vi "SubMark.vi"(0 "Refnum in":T1, 2 "Position Pixel":cluster{"x":sgl, "y":sgl}) -> ()   [LabVIEW 2015]
uses:
  <vilib>/vision/Image Controls.llb/IMAQ Image.ctl
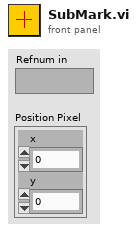
[diagram p1: front panel]
types:
  T1 = typedef "IMAQ Image.ctl" = refnum<image>
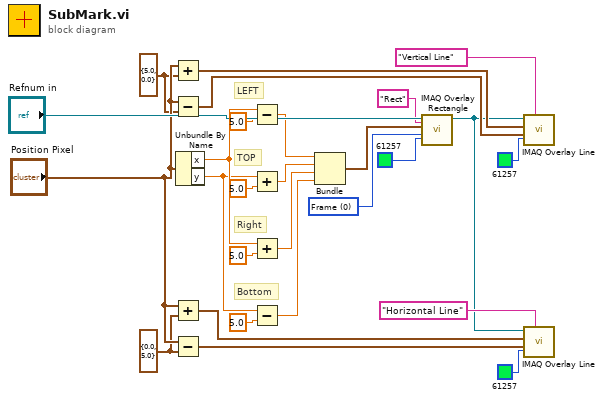
[diagram p0: block diagram]
diagram:
  w9 = cluster{"x":sgl, "y":sgl} {"x"=0.0, "y"=5.0} ("y")
  w14 = cluster{"x":sgl, "y":sgl} {"x"=5.0, "y"=0.0} ("y")
  w15 = u32 0 items=["Frame", "Fill", "Highlight"] ("Drawing Mode (Frame)")
  # "Bottom"
  # "Right"
  # "TOP"
  # "LEFT"
  n1 = Add(x="Position Pixel", y=w14) -> (x+y=w5:cluster{"x":sgl, "y":sgl})
  n2 = Subtract(x="Position Pixel", y=w14) -> (x-y=w13:cluster{"x":sgl, "y":sgl})
  n3 = Add(x="Position Pixel", y=w9) -> (x+y=w1:cluster{"x":sgl, "y":sgl})
  n4 = Subtract(x="Position Pixel", y=w9) -> (x-y=w8:cluster{"x":sgl, "y":sgl})
  n5 = Unbundle By Name("Position Pixel") -> ("x"=w3:sgl, "y"=w2:sgl)
  n6 = Subtract(x=w3, y=5.0) -> (x-y=w21:dbl)
  n7 = Add(x=w2, y=5.0) -> (x+y=w20:dbl)
  n8 = Add(x=w3, y=5.0) -> (x+y=w19:dbl)
  n9 = Subtract(x=w2, y=5.0) -> (x-y=w18:dbl)
  n10 = Bundle(w21, w20, w19, w18) -> (w17:cluster{dbl, dbl, dbl, dbl})  [unwired: 1 in]
  n11 = call "IMAQ Overlay Rectangle"("Color"=u32 61257, "Group"="Rect", "Drawing Mode (Frame)"=w15, "Rectangle"=w17, "Image"="Refnum in") -> ("Image Out"=w4:T1)  [unwired: 5 in, 1 out]
  n12 = call "IMAQ Overlay Line"("Color"=u32 61257, "Group"="Vertical Line", "End Point"=w13, "Start Point"=w5, "Image"=w4) -> ()  [unwired: 5 in, 2 out]
  n13 = call "IMAQ Overlay Line"("Color"=u32 61257, "Group"="Horizontal Line", "End Point"=w8, "Start Point"=w1, "Image"=w4) -> ()  [unwired: 5 in, 2 out]
